vi "Update.vi"(8 "error in (no error)":errorcluster) -> (0 "error out":errorcluster, 2 "Update":bool, 3 "UpdatePath":string)   [LabVIEW 2013, in "main.lvlib"]
uses:
  main.lvlib
  <userlib>/_MGI/Error Handling/MGI Suppress Error Code/MGI Suppress Error Code (Scalar).vi
panel:
  out "Update_TitleStr":string
  in  "Update_WaitMsgStr":string="Vent venligst mens opdateringen downloades..."
  in  "Update_SearchStr":string="Søg efter opdatering"
  in  "Update_CancelBtn":bool
  in  "Update_CurrentVerStr":string="Din nuværende version er: "
  in  "Update_LocateError":string="Fejl. Kunne ikke finde ny version."
  in  "Update_NetworkErrorStr":string="Netværksfejl. Bekræft forbindelsen"
  in  "Update_NewestVersionStr":string="Programmet er den nyeste version"
  in  "Update_NewVersionStr":string="Der er en ny opdatering til version: "
  out "String":string
  in  "UpdateProgram_btn":bool caption="UpdateProgram"
  out "VersionInformationStr":string
  in  "Update_CheckVersionsBtn":bool caption="CheckVersionsBtn"
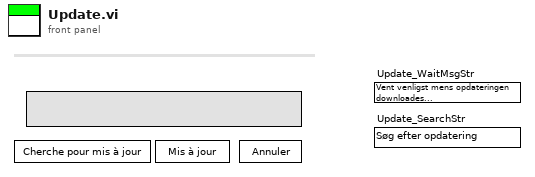
[diagram p1: front panel]
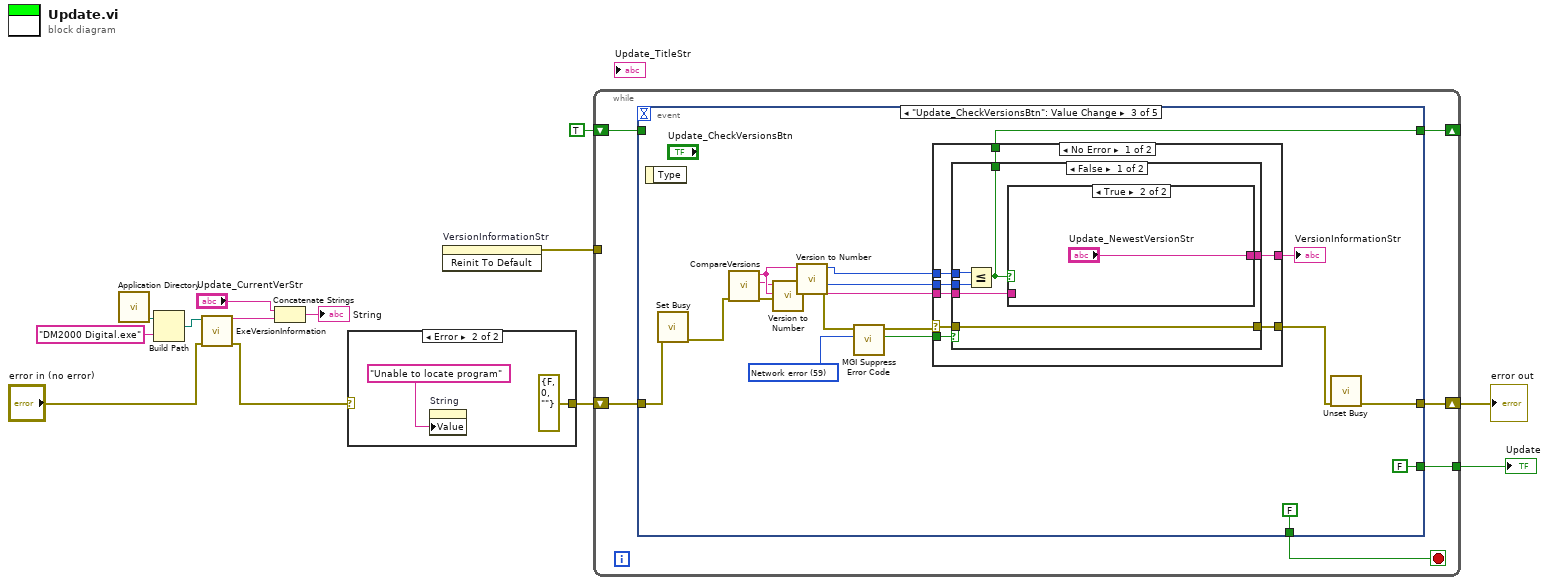
[diagram p0: block diagram]
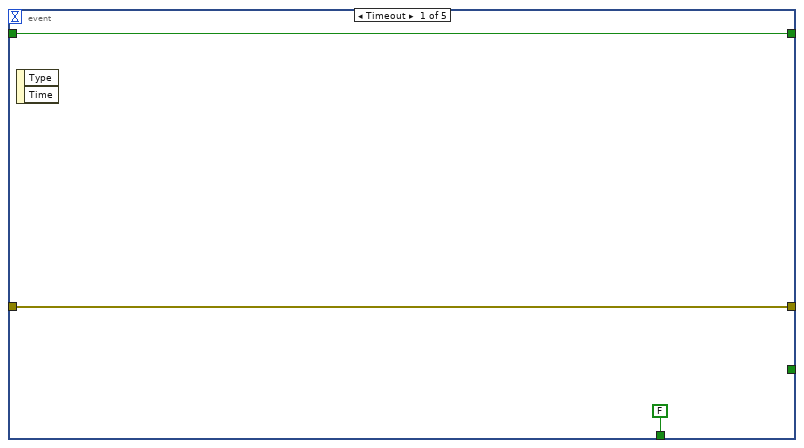
[diagram p3: hidden frame]
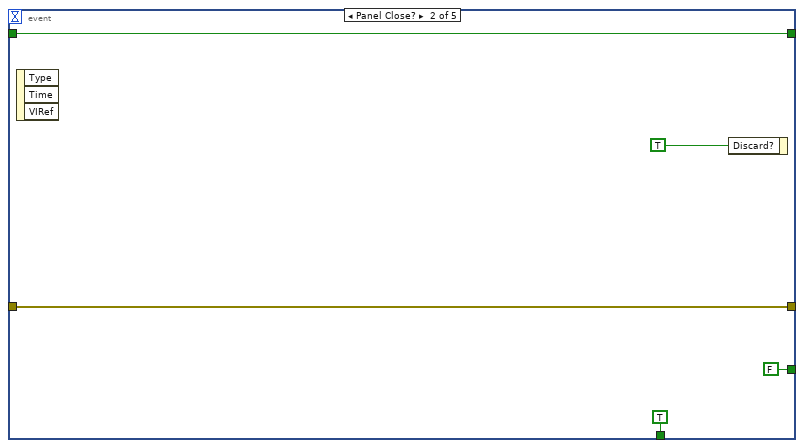
[diagram p4: hidden frame]
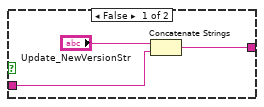
[diagram p5: hidden frame]
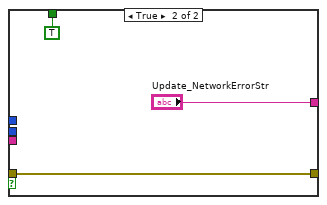
[diagram p6: hidden frame]
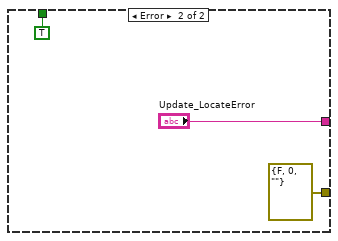
[diagram p7: hidden frame]
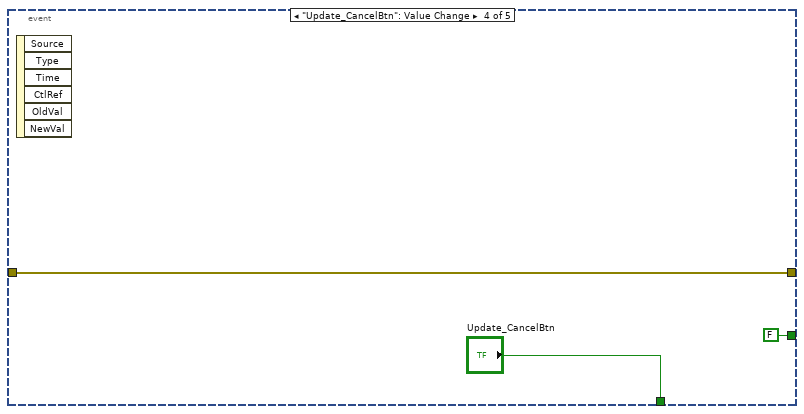
[diagram p8: hidden frame]
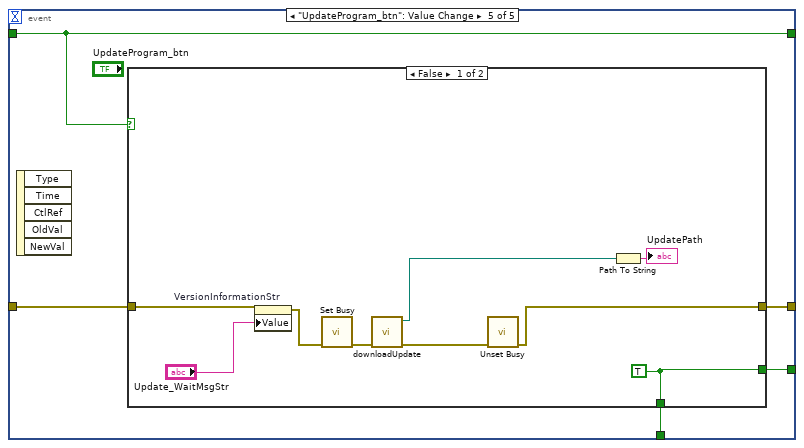
[diagram p9: hidden frame]
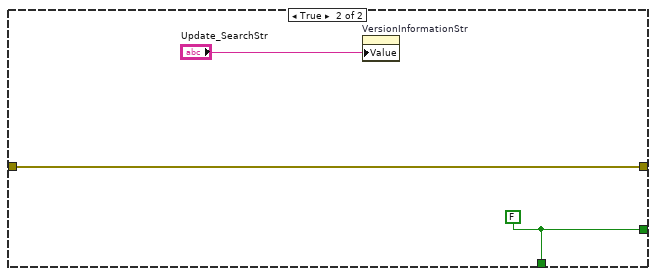
[diagram p10: hidden frame]
diagram:
  n1 = call <vilib>:"Application Directory.vi"() -> ("Application Directory"=w10:path)
  n2 = Build Path(base path=w10, name or relative path="DM2000 Digital.exe") -> (appended path=w8:path)
  n3 = call "ExeVersionInformation.vi"("error in (no error)"="error in (no error)", "path"=w8) -> ("error out"=w2:errorcluster, "FileVersion"=w6:string)  [unwired: 8 in]
  n4 = Concatenate Strings("Update_CurrentVerStr", w6) -> (→"String":string)
  n5 = case shown="Error" w2 {
    selector: w2 -> [w14 _]
    tunnel: [w14 errorcluster {"status"=FALSE, "code"=0, "source"=""} ("error IO")] -> w1
    frame No Error {
    }
    frame Error {
      n6 = property on="String" class="Str"("Value"="Unable to locate program" ("String")) -> ()  [unwired: 2 in, 2 out]
    }
  }
  n7 = invoke on="VersionInformationStr" class="Str" method="Reinit To Default"() -> (error out=w11:errorcluster)  [unwired: 3 in, 2 out]
  n8 = while {
    shift-right: [w21] -> _
    shift-left: TRUE -> [w20]
    tunnel: [w19] -> w12
    tunnel: w11 -> [_]
    shift-right: [w17] -> w4
    shift-left: w1 -> [w18]
    stop <- w22 stop-if-true
    n9 = event shown="[2] \"Update_CheckVersionsBtn\": Value Change" {
      selector: _ -> [_ _ _ _ _]
      dyn-events: _ -> [_ _ _ _ _]
      timeout: _ -> [_ _ _ _ _]
      tunnel: [FALSE TRUE FALSE "Update_CancelBtn" w79] -> w22
      tunnel: [w24 w28 w45 _ w80] -> w21
      tunnel: w20 -> [w24 w28 _ _ w80]
      tunnel: [_ FALSE FALSE FALSE w78] -> w19
      tunnel: w18 -> [w23 w26 w38 w73 w77]
      tunnel: [w23 w26 w37 w73 w76] -> w17
      event Timeout {
        n10 = event-data() -> ()  [unwired: 1 in, 2 out]
      }
      event Panel Close? {
        n11 = event-data() -> ()  [unwired: 1 in, 3 out]
        n12 = event-data("Discard?"=TRUE) -> ()  [unwired: 1 in, 1 out]
      }
      event "Update_CheckVersionsBtn": Value Change {
        w43 = 59 items=["No error", "Argument error", "Memory is full", "Out of zone", "End of file", "File already open", "Generic file I/O error", "File not found", "File permission error", "Disk is full", "Duplicate path", "Too many files open", "System feature not enabled", "Resource file not found", "Cannot add resource", "Resource not found", "Image not found", "Image memory error", "Pen does not exist", "Config type invalid", "Config token not found", "Config parse error", "Config memory error", "Bad external code format", "Bad external code offset", "External code not present", "Null window", "Destroy window error", "Null menu", "Print aborted", "Bad print record", "Print driver error", "Windows error during printing", "Memory error during printing", "Print dialog error", "Generic print error", "Invalid device refnum", "Device not found", "Device parameter error", "Device unit error", "Cannot open device", "Device call aborted", "Generic error", "Cancelled by user", "Object ID too low", "Object ID too high", "Object not in heap", "Unknown heap", "Unknown object (invalid DefProc)", "Unknown object (DefProc not in table)", "Message out of range", "Invalid (null) method", "Unknown message", "Manager call not supported", "Bad address", "Network operation in progress", "Network operation timed out", "Connection is busy", "Network attribute not supported", "Network error", "Address in use", "System out of memory", "Connection aborted", "Connection refused", "Not connected", "Already connected", "Connection closed", "Initialization error (interapplication manager)", "Bad occurrence", "Wait on unbound occurrence handler", "Occurrence queue overflow", "Datalog type conflict", "Unused", "Unrecognized type (interapplication manager)", "Memory corrupt", "Failed to make temporary DLL", "Old CIN version", "Drag socket not found", "Failed to load drop-object", "Failed to register OLE object", "Failed to release OLE object", "Format specifier type mismatch", "Unknown format specifier", "Too few format specifiers", "Too many format specifiers", "Scan failed", "Newer CIN version", "OLE Convert", "Runtime menu error", "Password tampered", "Unknown error code"] ("Error Code")
        n13 = event-data() -> ()  [unwired: 1 in, 1 out]
        n14 = call <vilib>:"Set Busy.vi"("error in (no error)"=w38) -> ("error out"=w46:errorcluster)  [unwired: 9 in, 1 out]
        n15 = call "CompareVersions.vi"("error in (no error)"=w46) -> ("error out"=w36:errorcluster, "FileVersion"=w40:string, "Web File Version"=w41:string)  [unwired: 8 in]
        n16 = call "Version to Number.vi"("error in"=w36, "Web File Version in"=w40) -> ("error out"=w35:errorcluster, "result"=w39:i32)  [unwired: 8 in]
        n17 = call "Version to Number.vi"("error in"=w35, "Web File Version in"=w41) -> ("error out"=w34:errorcluster, "result"=w33:i32)  [unwired: 8 in]
        n18 = call-poly <userlib>:"MGI Suppress Error Code.vi"("Error Code"=w43, "Error In"=w34) -> ("Error Supressed?"=w42:bool, "Error Out"=w32:errorcluster)  [unwired: 4 in]
        n19 = case shown="No Error" w32 {
          selector: w32 -> [w50 _]
          tunnel: [w56 "Update_LocateError"] -> w47
          tunnel: [w55 TRUE] -> w45
          tunnel: w42 -> [w54 _]
          tunnel: w41 -> [w53 _]
          tunnel: w39 -> [w52 _]
          tunnel: w33 -> [w51 _]
          tunnel: [w49 errorcluster {"status"=FALSE, "code"=0, "source"=""} ("error IO")] -> w31
          frame No Error {
            n20 = case shown="False" w54 {
              tunnel: [w62 "Update_NetworkErrorStr"] -> w56
              tunnel: [w61 TRUE] -> w55
              tunnel: w53 -> [w60 _]
              tunnel: w51 -> [w59 _]
              tunnel: w52 -> [w58 _]
              tunnel: w50 -> [w57 w67]
              tunnel: [w57 w67] -> w49
              frame False {
                n21 = Less Or Equal?(x=w59, y=w58) -> (x <= y?=w61:bool)
                n22 = case shown="True" w61 {
                  tunnel: [w65 "Update_NewestVersionStr"] -> w62
                  tunnel: w60 -> [w63 _]
                  frame False {
                    n23 = Concatenate Strings("Update_NewVersionStr", w63) -> (w65:string)
                  }
                  frame True {
                  }
                }
              }
              frame True {
              }
            }
          }
          frame Error {
          }
        }
        "VersionInformationStr" <- w47
        n24 = call <vilib>:"Unset Busy.vi"("error in (no error)"=w31) -> ("error out"=w37:errorcluster)  [unwired: 10 in]
      }
      event "Update_CancelBtn": Value Change {
        n25 = event-data() -> ()  [unwired: 1 in, 6 out]
      }
      event "UpdateProgram_btn": Value Change {
        n26 = event-data() -> ()  [unwired: 1 in, 5 out]
        n27 = case shown="False" w80 {
          tunnel: [w86 w91] -> w79
          tunnel: [w86 w91] -> w78
          tunnel: w77 -> [w82 w90]
          tunnel: [w81 w90] -> w76
          frame False {
            w86 = TRUE
            n28 = property on="VersionInformationStr" class="Str"(error in=w82, "Value"="Update_WaitMsgStr") -> (error out=w88:errorcluster)  [unwired: 1 in, 1 out]
            n29 = call <vilib>:"Set Busy.vi"("error in (no error)"=w88) -> ("error out"=w85:errorcluster)  [unwired: 9 in, 1 out]
            n30 = call "downloadUpdate.vi"("error in (no error)"=w85) -> ("error out"=w83:errorcluster, "appended path"=w84:path)  [unwired: 9 in]
            n31 = call <vilib>:"Unset Busy.vi"("error in (no error)"=w83) -> ("error out"=w81:errorcluster)  [unwired: 10 in]
            n32 = Path To String(path=w84) -> (string=→"UpdatePath":string)
          }
          frame True {
            w91 = FALSE
            n33 = property on="VersionInformationStr" class="Str"("Value"="Update_SearchStr") -> ()  [unwired: 2 in, 2 out]
          }
        }
      }
    }
  }
  "Update" <- w12
  "error out" <- w4
